vi "A Alignment.vi"(10 "Potentiometer Value":dbl) -> ()   [LabVIEW 2015]
uses:
  <vilib>/Rock Robotics/WPI/CAN/TalonSRX/WPI_CANTalonSRX_APIControlMode.ctl
  <vilib>/Rock Robotics/WPI/Solenoid/WPI_SolenoidValue.ctl
  <vilib>/Rock Robotics/WPI/Utilities/WPI_GetSetVariantRefNum.vi
  Robot Global Data.vi
  <vilib>/Rock Robotics/WPI/Solenoid/WPI_SolenoidSetEnum.vi
panel:
  in  "Turn Speed":dbl=0.35
  out "x":dbl
  in  "Shooting RPM":dbl=2500.0
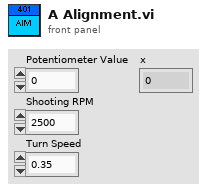
[diagram p1: front panel]
types:
  T1 = enum16{"Horizontal Aiming", "Shoot", "End", "Spin Shooter", "Vertical Aiming"}
  T2 = typedef "WPI_MotorControlDeviceRef.ctl" = cluster{"DeviceStatus":errorcluster, "Type":T3, "PWM":cluster{"PWM Channel":T4, "DeadBand":T5}, "CAN":cluster{"Device Number":u8, "Control Mode":T6, "Semaphore":T7, "Max Vout":dbl, "TalonSRX Control Mode":T8}, "Invert":bool}
  T3 = typedef "WPI_MotorControlType.ctl" = enum16{"PWM", "CAN", "CANTalonSRX"}
  T4 = typedef "FPGA_DIOPWMChannel.ctl" = enum8{"PWM 0", "PWM 1", "PWM 2", "PWM 3", "PWM 4", "PWM 5", "PWM 6", "PWM 7", "PWM 8", "PWM 9", "PWM MXP 0", "PWM MXP 1", "PWM MXP 2", "PWM MXP 3", "PWM MXP 4", "PWM MXP 5", "PWM MXP 6", "PWM MXP 7", "PWM MXP 8", "PWM MXP 9", "Invalid"}
  T5 = typedef "WPI_PWMDeadband.ctl" = cluster{"Name":string, "maxPositivePwm":i32, "minPositivePwm":i32, "centerPwm":i32, "maxNegativePwm":i32, "minNegativePwm":i32, "angularRange":u16}
  T6 = typedef "WPI_CANJaguar_ControlMode.ctl" = enum8{"Percent VBus", "Current", "Speed", "Position", "Voltage"}
  T7 = typedef "Semaphore RefNum" = refnum<k1>
  T8 = typedef "WPI_CANTalonSRX_APIControlMode.ctl" = enum8{"Percent VBus", "Speed", "Position", "Slave", "Unchanged / Invalid", "Voltage Compensation", "Current", "Motion Profile"}
  T9 = typedef "WPI_RobotDriveDevRef.ctl" = cluster{"DevStatus":errorcluster, "Motors[]":T2[], "Square Inputs":bool, "Max Output":dbl}
  T10 = typedef "WPI_SolenoidDevRef.ctl" = cluster{"DevStatus":errorcluster, "Pneumatics Control Module":u8, "Forward Solenoid Channel":T11, "Reverse Solenoid Channel":T11}
  T11 = typedef "WPI_SolenoidChannel.ctl" = enum8{"Solenoid 0", "Solenoid 1", "Solenoid 2", "Solenoid 3", "Solenoid 4", "Solenoid 5", "Solenoid 6", "Solenoid 7", "Invalid"}
  T12 = typedef "WPI_SolenoidValue.ctl" = enum16{"Off", "On", "Forward", "Reverse"}
  T13 = typedef "WPI_CANTalonSRX_GlobalStatus.ctl" = cluster{"Applied Throttle":dbl, "Module Enabled":bool, "CAN Error":errorcluster, "Closed Loop Error":dbl, "Forward Limit Switch Closed":bool, "Reverse Limit Switch Closed":bool, "Sensor Position":dbl, "Sensor Velocity":dbl, "Current":dbl, "Sticky Fault - Over Temp":bool, "Sticky Fault - Under Voltage":bool, "Sticky Fault - Forward Limit":bool, "Sticky Fault - Reverse Limit":bool, "Sticky Fault - Forward Soft Limit":bool, "Sticky Fault - Reverse Soft Limit":bool, "Brake is Enabled":bool, "Encoder Position":dbl, "Encoder Velocity":dbl, "Encoder Index Count":dbl, "Encoder A Pin State":bool, "Encoder B Pin State":bool, "Encoder Index Pin State":bool, "Analog In":dbl, "Analog In Velocity":dbl, "Temperature (C)":dbl, "Battery Voltage":dbl, "Control 5 Is Supported":bool, "Current Profile Slot Select":dbl, "Pos Div 8":bool, "Vel Div 4":bool, "Pulse Width Position":i32, "Pulse Width Velocity":i32, "Pulse Width Rise To Rise (us)":i32, "Pulse Width Rise To Fall (us)":i32, "Mot Prof Active Is Under Run":bool, "Mot Prof Active Has Under Run":bool, "Mot Prof Active Is Last":bool, "Mot Prof Active Velocity Only":bool, "Mot Prof Active Is Valid":bool, "Mot Prof Buffer Is Full":bool, "Mot Prof Active Profile Slot Select":i32, "Mot Prof NextID":i32, "Mot Prof Count":i32, "Mot Prof Active Velocity":dbl, "Mot Prof Active Position":dbl, "Mot Prof Output Enable":i32}
  T14 = cluster{"y":dbl, "Distance":dbl, "Angle":dbl, "Goal?":bool, "x":dbl}
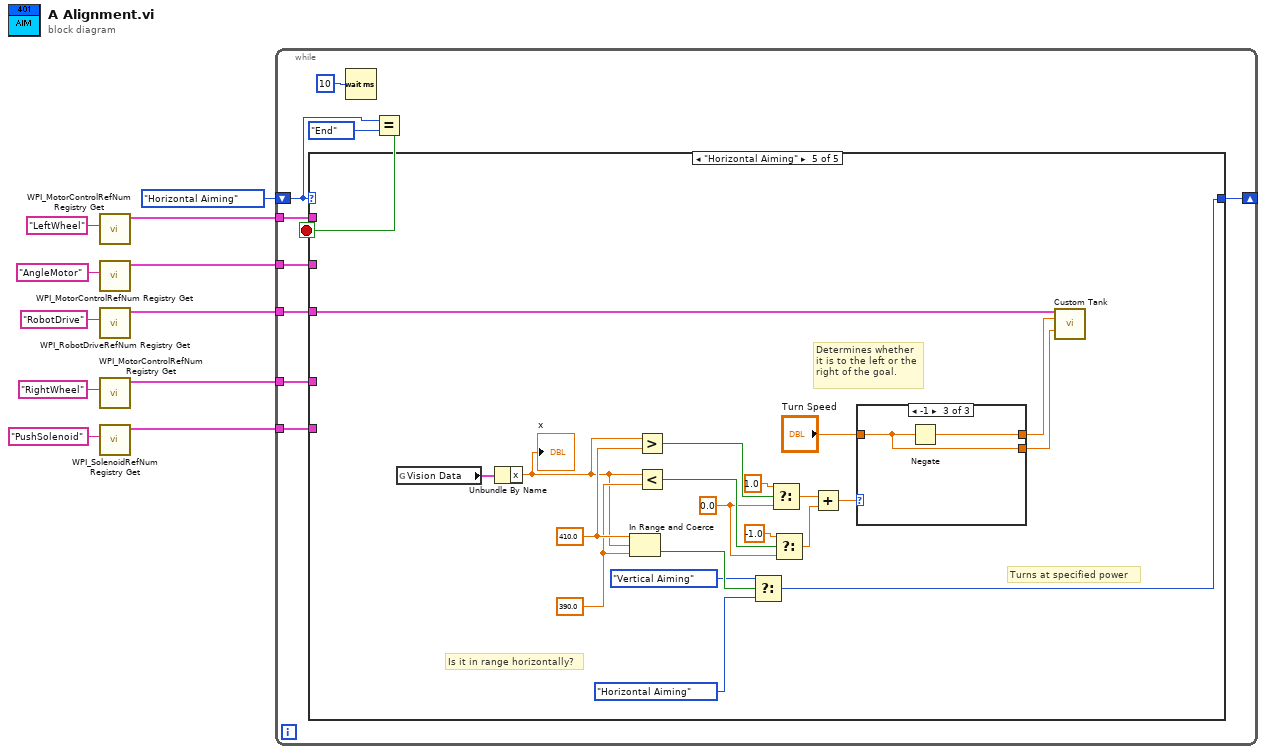
[diagram p0: block diagram]
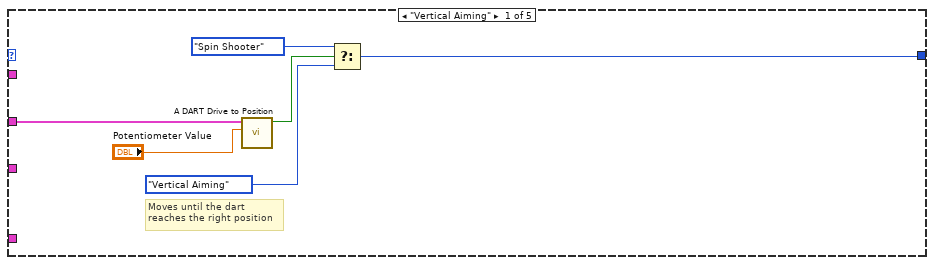
[diagram p2: hidden frame]
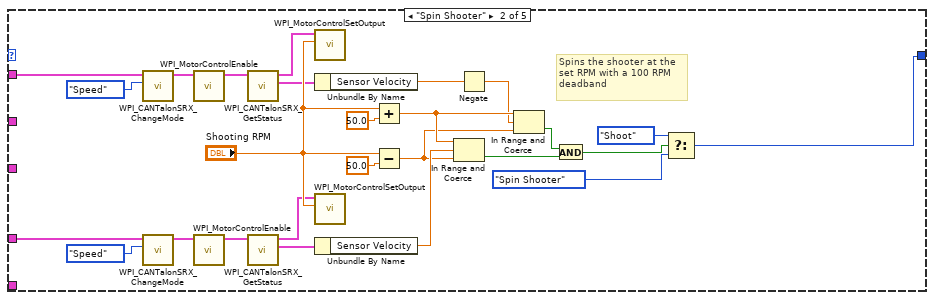
[diagram p3: hidden frame]
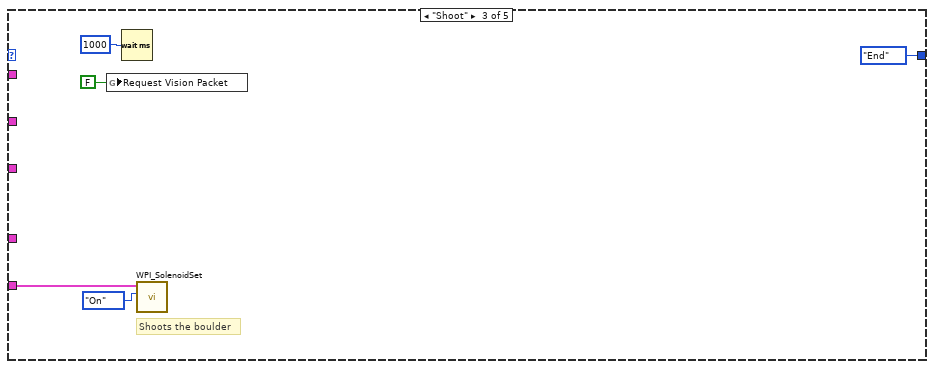
[diagram p4: hidden frame]
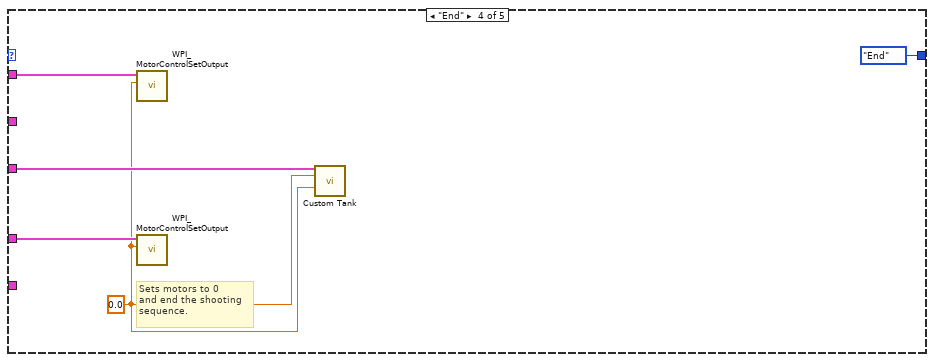
[diagram p5: hidden frame]
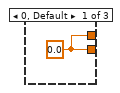
[diagram p6: hidden frame]
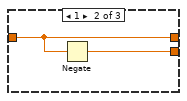
[diagram p7: hidden frame]
diagram:
  n1 = call <vilib>:"WPI_MotorControlRefNum Registry Get.vi"("refnum name"="LeftWheel") -> ("MotorControlDevRef"=w9:T2)  [unwired: 9 in, 1 out]
  n2 = call <vilib>:"WPI_MotorControlRefNum Registry Get.vi"("refnum name"="AngleMotor") -> ("MotorControlDevRef"=w10:T2)  [unwired: 9 in, 1 out]
  n3 = call <vilib>:"WPI_RobotDriveRefNum Registry Get.vi"("refnum name"="RobotDrive") -> ("RobotDriveDevRef"=w11:T9)  [unwired: 9 in, 1 out]
  n4 = call <vilib>:"WPI_MotorControlRefNum Registry Get.vi"("refnum name"="RightWheel") -> ("MotorControlDevRef"=w8:T2)  [unwired: 9 in, 1 out]
  n5 = call <vilib>:"WPI_SolenoidRefNum Registry Get.vi"("refnum name"="PushSolenoid") -> ("SolenoidDevRef"=w7:T10)  [unwired: 9 in, 1 out]
  n6 = while {
    tunnel: w11 -> [w21]
    shift-right: [w20] -> _
    shift-left: T1."Horizontal Aiming" -> [w13]
    tunnel: w10 -> [w19]
    tunnel: w9 -> [w18]
    tunnel: w8 -> [w17]
    tunnel: w7 -> [w16]
    stop <- w12 stop-if-true
    n7 = case shown="\"Horizontal Aiming\"" w13 {
      tunnel: w21 -> [_ _ _ w60 w81]
      tunnel: [w22 w28 T1."End" T1."End" w79] -> w20
      tunnel: w19 -> [w27 _ _ _ _]
      tunnel: w18 -> [_ w50 _ w61 _]
      tunnel: w17 -> [_ w49 _ w62 _]
      tunnel: w16 -> [_ _ w57 _ _]
      frame "Vertical Aiming" {
        # "Moves until the dart\nreaches the right position"
        n8 = call "A DART Drive to Position.vi"("Potentiometer Value"="Potentiometer Value", "MotorControlDevRef"=w27) -> ("Boolean"=w23:bool)  [unwired: 9 in]
        n9 = Select(t=T1."Spin Shooter", s=w23, f=T1."Vertical Aiming") -> (s? t:f=w22:T1)
      }
      frame "Spin Shooter" {
        # "Spins the shooter at the \nset RPM with a 100 RPM\ndeadband"
        n10 = call <vilib>:"WPI_CANTalonSRX_ChangeMode.vi"("Control Mode"=WPI_CANTalonSRX_APIControlMode."Speed", "CAN Talon SRX Ref"=w50) -> ("CAN Talon SRX Ref"=w48:T2)  [unwired: 8 in, 1 out]
        n11 = call <vilib>:"WPI_CANTalonSRX_ChangeMode.vi"("Control Mode"=WPI_CANTalonSRX_APIControlMode."Speed", "CAN Talon SRX Ref"=w49) -> ("CAN Talon SRX Ref"=w52:T2)  [unwired: 8 in, 1 out]
        n12 = call <vilib>:"WPI_MotorControlEnable.vi"("CAN MotorDevRef"=w48) -> ("CAN MotorDevRef"=w45:T2)  [unwired: 9 in, 1 out]
        n13 = call <vilib>:"WPI_MotorControlEnable.vi"("CAN MotorDevRef"=w52) -> ("CAN MotorDevRef"=w46:T2)  [unwired: 9 in, 1 out]
        n14 = call <vilib>:"WPI_CANTalonSRX_GetStatus.vi"("CAN Talon SRX Ref"=w45) -> ("Talon SRX Status"=w44:T13, "CAN Talon SRX Ref"=w35:T2)  [unwired: 8 in, 1 out]
        n15 = call <vilib>:"WPI_CANTalonSRX_GetStatus.vi"("CAN Talon SRX Ref"=w46) -> ("Talon SRX Status"=w43:T13, "CAN Talon SRX Ref"=w34:T2)  [unwired: 8 in, 1 out]
        n16 = call <vilib>:"WPI_MotorControlSetOutput.vi"("Output"="Shooting RPM", "MotorControlDevRef"=w35) -> ()  [unwired: 7 in, 3 out]
        n17 = Unbundle By Name(w44) -> ("Sensor Velocity"=w33:dbl)
        n18 = call <vilib>:"WPI_MotorControlSetOutput.vi"("Output"="Shooting RPM", "MotorControlDevRef"=w34) -> ()  [unwired: 7 in, 3 out]
        n19 = Unbundle By Name(w43) -> ("Sensor Velocity"=w42:dbl)
        n20 = Add(x="Shooting RPM", y=50.0) -> (x+y=w39:dbl)
        n21 = Subtract(x="Shooting RPM", y=50.0) -> (x-y=w38:dbl)
        n22 = In Range and Coerce(upper limit=w39, x=w42, lower limit=w38) -> (In Range?=w36:bool)  [unwired: 1 out]
        n23 = Negate(x=w33) -> (-x=w32:dbl)
        n24 = In Range and Coerce(upper limit=w39, x=w32, lower limit=w38) -> (In Range?=w37:bool)  [unwired: 1 out]
        n25 = And(x=w37, y=w36) -> (x .and. y?=w29:bool)
        n26 = Select(t=T1."Shoot", s=w29, f=T1."Spin Shooter") -> (s? t:f=w28:T1)
      }
      frame "Shoot" {
        # "Shoots the boulder"
        n27 = global write "Robot Global Data.vi" "Request Vision Packet"(FALSE) -> ()
        n28 = Wait (ms)(milliseconds to wait=u32 1000) -> ()  [unwired: 1 out]
        n29 = call-poly <vilib>:"WPI_SolenoidSet.vi"("Value"=WPI_SolenoidValue."On", "SolenoidDevRef"=w57) -> ()  [unwired: 8 in, 2 out]
      }
      frame "End" {
        w59 = 0.0 ("Left axis value")
        # "Sets motors to 0\nand end the shooting\nsequence."
        n30 = call <vilib>:"WPI_MotorControlSetOutput.vi"("Output"=w59, "MotorControlDevRef"=w61) -> ()  [unwired: 7 in, 3 out]
        n31 = call <vilib>:"WPI_MotorControlSetOutput.vi"("Output"=w59, "MotorControlDevRef"=w62) -> ()  [unwired: 7 in, 3 out]
        n32 = call "Custom Tank.vi"("RobotDriveDevRef 2"=w60, "Left axis value"=w59, "Right axis value"=w59) -> ()  [unwired: 8 in, 5 out]
      }
      frame "Horizontal Aiming" {
        w73 = 0.0 ("f")
        w82 = 390.0 ("lower limit")
        w83 = 410.0 ("upper limit")
        # "Turns at specified power"
        # "Determines whether\nit is to the left or the\nright of the goal."
        # "Is it in range horizontally?"
        n33 = global read "Robot Global Data.vi" "Vision Data"() -> (w64:T14)
        n34 = Unbundle By Name(w64) -> ("x"=w78:dbl)
        "x" <- w78
        n35 = In Range and Coerce(upper limit=w83, x=w78, lower limit=w82) -> (In Range?=w80:bool)  [unwired: 1 out]
        n36 = Greater?(x=w78, y=w83) -> (0:w77:bool)
        n37 = Less?(x=w78, y=w82) -> (x < y?=w76:bool)
        n38 = Select(t=T1."Vertical Aiming", s=w80, f=T1."Horizontal Aiming") -> (s? t:f=w79:T1)
        n39 = Select(t=1.0, s=w77, f=w73) -> (s? t:f=w72:dbl)
        n40 = Select(t=-1.0, s=w76, f=w73) -> (s? t:f=w71:dbl)
        n41 = Add(x=w72, y=w71) -> (x+y=w70:dbl)
        n42 = case shown="-1" w70 {
          tunnel: [w84 w86 w87] -> w69
          tunnel: [w84 w85 w88] -> w68
          tunnel: "Turn Speed" -> [_ w85 w87]
          frame 0, Default {
            w84 = 0.0
          }
          frame 1 {
            n43 = Negate(x=w85) -> (-x=w86:dbl)
          }
          frame -1 {
            n44 = Negate(x=w87) -> (-x=w88:dbl)
          }
        }
        n45 = call "Custom Tank.vi"("RobotDriveDevRef 2"=w81, "Left axis value"=w68, "Right axis value"=w69) -> ()  [unwired: 8 in, 5 out]
      }
    }
    n46 = Wait (ms)(milliseconds to wait=u32 10) -> ()  [unwired: 1 out]
    n47 = Equal?(x=w13, y=T1."End") -> (x = y?=w12:bool)
  }
